vi "Alpha 3.vi"() -> ()   [LabVIEW 2011]
uses:
  <vilib>/vision/NI_Vision_Development_Module.lvlib
panel:
  in  "Operation":T1(ring)
  in  "Square/Hexa":bool
  out "Contour Line":T2(plugin-control)
  in  "Threshold":cluster{u8, u8}(slide)={0, 6} scale=0.0..256.0
  in  "Stop":bool
  in  "Browse":bool
  out "Original Image":T2(plugin-control)
  out "Path to Image":path
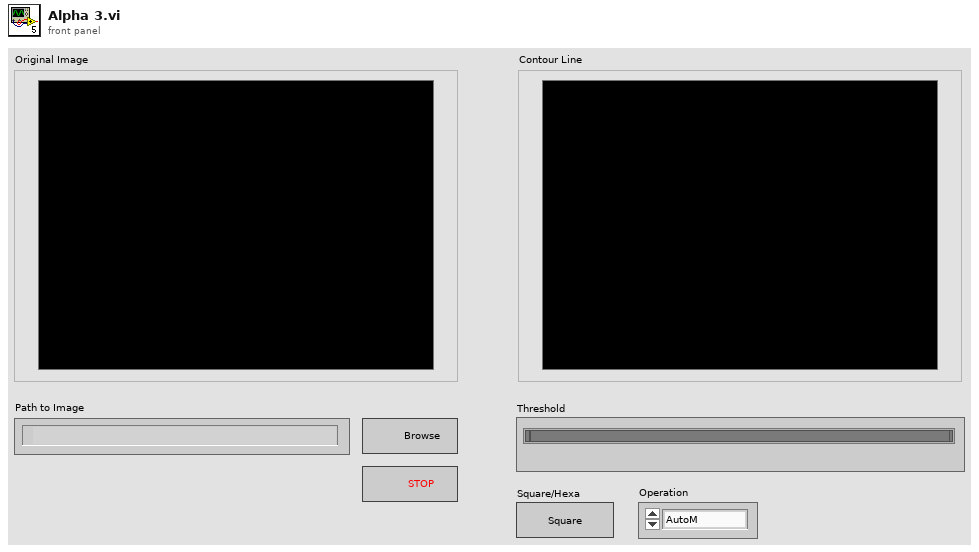
[diagram p1: front panel]
types:
  T1 = enum16{"AutoM", "Close", "Dilate", "Erode", "Gradient", "Gradient out", "Gradient in", "Hit miss", "Open", "PClose", "POpen", "Thick", "Thin"}
  T2 = typedef "IMAQ Image.ctl" = refnum<image>
  T3 = typedef "Image Type" = u32
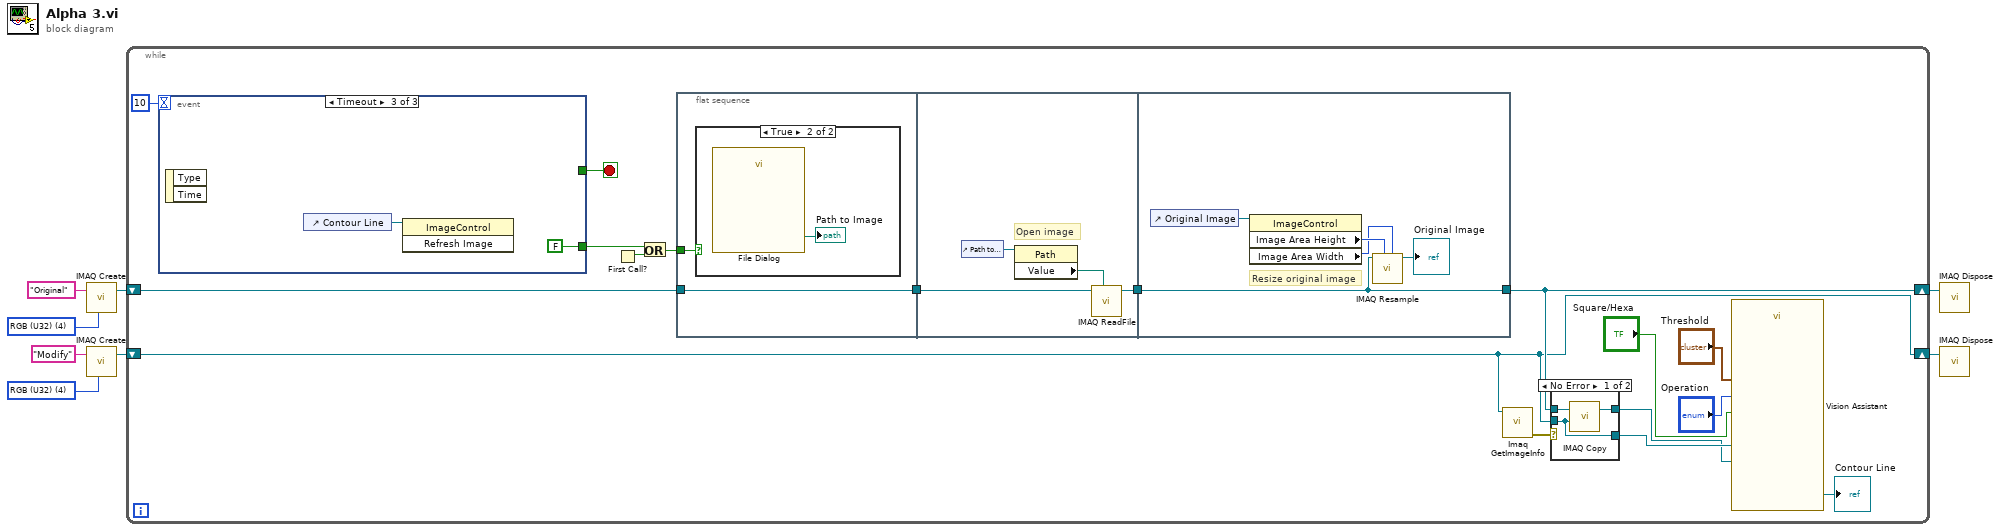
[diagram p0: block diagram]
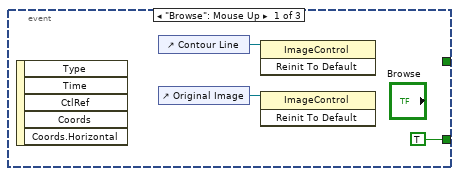
[diagram p4: hidden frame]
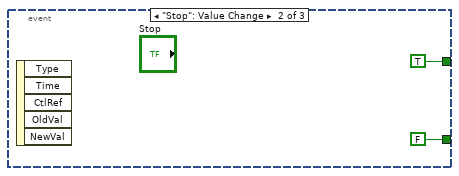
[diagram p5: hidden frame]
diagram:
  w1 = T3 4 items=["Grayscale (U8)", "Grayscale (I16)", "Grayscale (SGL)", "Complex (CSG)", "RGB (U32)", "HSL (U32)", "RGB (U64)", "Grayscale (U16)"] ("Image Type")
  w4 = T3 4 items=["Grayscale (U8)", "Grayscale (I16)", "Grayscale (SGL)", "Complex (CSG)", "RGB (U32)", "HSL (U32)", "RGB (U64)", "Grayscale (U16)"] ("Image Type")
  n1 = call "IMAQ Create"("Image Name"="Original", "Image Type"=w4) -> ("New Image"=w7:T2)  [unwired: 3 in, 1 out]
  n2 = call "IMAQ Create"("Image Name"="Modify", "Image Type"=w1) -> ("New Image"=w5:T2)  [unwired: 3 in, 1 out]
  n3 = while {
    shift-right: [w19] -> w3
    shift-left: w7 -> [w11]
    shift-right: [w18] -> w2
    shift-left: w5 -> [w18]
    stop <- w20 stop-if-true
    n4 = event shown="[2] Timeout" {
      selector: _ -> [_ _ _]
      dyn-events: _ -> [_ _ _]
      timeout: 10 -> [_ _ _]
      tunnel: [_ TRUE _] -> w20
      tunnel: [TRUE FALSE FALSE] -> w16
      event "Browse": Mouse Up {
        n5 = event-data() -> ()  [unwired: 1 in, 5 out]
        n6 = control-ref of="Contour Line"() -> (w45:refnum<vi>)
        n7 = control-ref of="Original Image"() -> (w44:refnum<vi>)
        n8 = invoke class="ImageControl" method="Reinit To Default"(reference=w45) -> ()  [unwired: 2 in, 3 out]
        n9 = invoke class="ImageControl" method="Reinit To Default"(reference=w44) -> ()  [unwired: 2 in, 3 out]
      }
      event "Stop": Value Change {
        n10 = event-data() -> ()  [unwired: 1 in, 5 out]
      }
      event Timeout {
        n11 = event-data() -> ()  [unwired: 1 in, 2 out]
        n12 = control-ref of="Contour Line"() -> (w49:refnum<vi>)
        n13 = invoke class="ImageControl" method="Refresh Image"(reference=w49) -> ()  [unwired: 2 in, 3 out]
      }
    }
    n14 = First Call?() -> (First Call?: T/F=w15:bool)
    n15 = Or(x=w16, y=w15) -> (x .or. y?=w12:bool)
    n16 = flat-sequence {
      tunnel: w12 -> [w32]
      tunnel: w11 -> [w31]
      tunnel: [w31] -> w10
      tunnel: [w37] -> w25
      tunnel: w10 -> [w34]
      tunnel: w25 -> [w38]
      tunnel: [w38] -> w19
      frame #0 {
        n17 = case shown="True" w32 {
          frame False {
          }
          frame True {
            n18 = call "File Dialog"() -> ("selected path"=→"Path to Image":path)  [unwired: 12 in, 3 out]
          }
        }
      }
      frame #1 {
        # "Open image"
        n19 = control-ref of="Path to Image"() -> (w36:refnum<vi>)
        n20 = property class="Path"(reference=w36) -> ("Value"=w35:path)  [unwired: 1 in, 2 out]
        n21 = call "IMAQ ReadFile"("File Path"=w35, "Image"=w34) -> ("Image Out"=w37:T2)  [unwired: 5 in, 4 out]
      }
      frame #2 {
        # "Resize original image"
        n22 = control-ref of="Original Image"() -> (w42:refnum<vi>)
        n23 = property class="ImageControl"(reference=w42) -> ("Image Area Height"=w41:u32, "Image Area Width"=w40:u32)  [unwired: 1 in, 2 out]
        n24 = call "IMAQ Resample"("X Resolution"=w40, "Y Resolution"=w41, "Image Src"=w38) -> ("Image Dst Out"=→"Original Image":T2)  [unwired: 7 in, 1 out]
      }
    }
    n25 = call "Imaq GetImageInfo"("Image"=w18) -> ("error out"=w24:errorcluster)  [unwired: 1 in, 9 out]
    n26 = case shown="No Error" w24 {
      tunnel: w18 -> [w26 w29]
      tunnel: [w28 w30] -> w22
      tunnel: w19 -> [w27 w30]
      tunnel: [w26 w29] -> w23
      frame No Error {
        n27 = call "IMAQ Copy"("Image Dst"=w26, "Image Src"=w27) -> ("Image Dst Out"=w28:T2)  [unwired: 4 in, 1 out]
      }
      frame Error {
      }
    }
    n28 = call "Vision Assistant"("Image In"=w22, "Image Dst"=w23, "Range (Threshold)"="Threshold", "Operation (Basic Morphology)"="Operation", "Square/Hexa (Square) (Basic Morphology)"="Square/Hexa") -> ("Image Out"=→"Contour Line":T2)  [unwired: 21 in, 1 out]
  }
  n29 = call "IMAQ Dispose"("Image"=w3) -> ()  [unwired: 5 in, 1 out]
  n30 = call "IMAQ Dispose"("Image"=w2) -> ()  [unwired: 5 in, 1 out]
